vi "Play Sound Tone.vi"() -> ()   [LabVIEW 2021]
uses:
  Globals/Meas_global.vi
  Globals/Trav_pos_global.vi
  Controls/Post_Process.ctl
  Controls/Setup.ctl
panel:
  out "Comments":string
  in  "device ID":u32
  # "Put in command file row comments: \n\nDesired Freq (Hz); Volume (%);\n\nExample\n\n500; 30;"
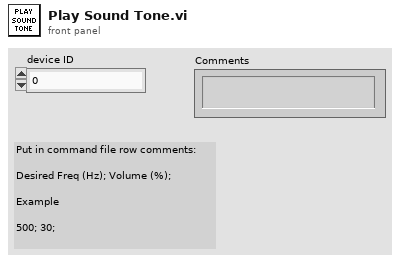
[diagram p1: front panel]
types:
  T1 = typedef "Setup.ctl" = enum16{"Run Program", "Show Setup", "Save Current Setup", "Setup Front Panel"}
  T2 = typedef "Post_Process.ctl" = enum16{"Take New Data", "Post Process Raw Data File"}
  T3 = typedef "Traverse_cluster.ctl" = cluster{"Start X":sgl, "Start Y":sgl, "Start Z":sgl, "End X":sgl, "End Y":sgl, "End Z":sgl, "nPoints":i32, "Spacing":T4, "Filename":path, "Tunnel Speed":dbl, "Averaging time (mins)":dbl, "Extra Commands":string, "Carrier_1 Q (l/min)":dbl, "Carrier_2 Q (l/min)":dbl, "Trace Gas Concentration (%)":dbl, "Specific Arguments":string, "Comments":string, "Row No":i32, "Row Type Selector":T5, "EstCompl":string, "Row Duration (mins)":dbl, "nValidPoints":i32, "Meas Setup File":string}
  T4 = typedef "Spacing.ctl" = enum16{"Linear", "Log", "Gauss", "Specified", "N/A"}
  T5 = typedef "Multi_run_mode.ctl" = enum16{"Move Traverse Only", "Set Tunnel Speed Only", "Set Source Only", "Set Measurement Conditions", "Single Measurement", "Vertical Profile", "Lateral Profile", "Longitudinal Profile", "Multi-Axis Profile", "Explore Volume", "Auto Calibrate", "Meas Fast FID Bkgnd", "Check Beam Power", "Scanning Valve Measurement", "Run VI Named:", "Set ADAM Ch", "Wait (minutes)", "Send Message", "Synchronize With:", "Fall Back to this Row", "Turn Off Row Repeating", "Traverse 3D Volume", "Blank Row", "Jump to Fall Back Row"}
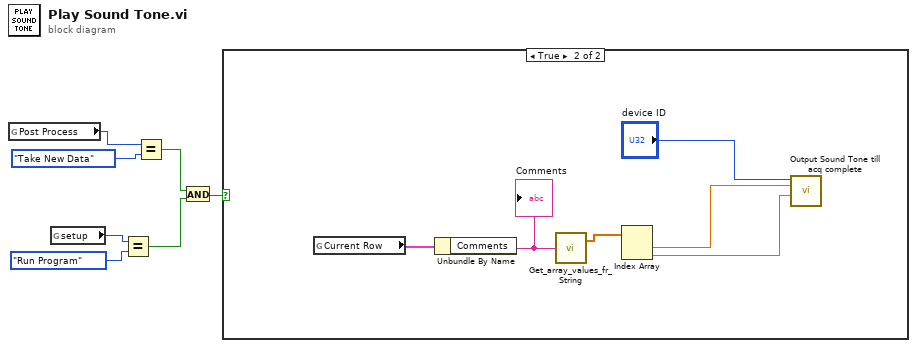
[diagram p0: block diagram]
diagram:
  n1 = global read "Meas_global.vi" "Post Process"() -> (w4:T2)
  n2 = global read "Meas_global.vi" "setup"() -> (w6:T1)
  n3 = Equal?(x=w6, y=Setup."Run Program" ("setup")) -> (x = y?=w3:bool)
  n4 = Equal?(x=w4, y=Post_Process."Take New Data" ("Post Process")) -> (x = y?=w2:bool)
  n5 = And(x=w2, y=w3) -> (x .and. y?=w1:bool)
  n6 = case shown="True" w1 {
    frame False {
    }
    frame True {
      n7 = global read "Trav_pos_global.vi" "Current Row"() -> (w12:T3)
      n8 = Unbundle By Name(w12) -> ("Comments"=w11:string)
      "Comments" <- w11
      n9 = call "Get_array_values_fr_String.vi"("String Value"=w11) -> ("Numeric Array"=w10:dbl[])  [unwired: 1 out]
      n10 = Index Array(array=w10) -> (element #1=w9:dbl, element #2=w8:dbl)  [unwired: 2 in]
      n11 = call "Output Sound Tone till acq complete.vi"("device ID"="device ID", "frequency"=w9, "volume"=w8) -> ()  [unwired: 4 in, 1 out]
    }
  }
